vi "host.vi"() -> ()   [LabVIEW 2020]
uses:
  <vilib>/Analysis/baseanly.llb/Vector x A.vi
  <vilib>/Analysis/baseanly.llb/Real Dot Product.vi
  <vilib>/Analysis/Matrix/Numeric/Conversions/Array To Matrix - RA2.vi
  <vilib>/FPGAPlugInAG/cRIO-9054/niLvFpga_Open_cRIO-9054.vi
  <vilib>/rvi/interface/common/dynamic/niFpgaDynamicAddResources.vi
  <vilib>/Utility/error.llb/Error Cluster From Error Code.vi
  <vilib>/rvi/errors/niLvFpgaAdjustHostInterfaceError.vi
  <vilib>/FPGAPlugInAG/Dynamic/niLvFpga_Run_Dynamic.vi
  <vilib>/FPGAPlugInAG/Dynamic/niLvFpga_Close_Dynamic.vi
  <vilib>/rvi/interface/nirviOpenFPGA/nirviOpenFPGA.xnode
  FPGA Bitfiles/mlpsizing_FPGATarget_target_1fQeBnJI5tw.lvbitx
  target.vi
  <vilib>/rvi/interface/nirviMethod/nirviMethod.xnode
  <vilib>/rvi/interface/nirviReadWriteControl/nirviReadWriteControl.xnode
  <vilib>/rvi/interface/nirviCloseFPGA/nirviCloseFPGA.xnode
  <vilib>/Analysis/NI_AALBase.lvlib
  <vilib>/Analysis/Matrix/NI_Matrix.lvlib
  <vilib>/FPGAPlugInAG/Dynamic/niLvFpga_WriteFifo_Dynamic.vi
  <vilib>/rvi/errors/niLvFpgaMergeErrorWithErrorCode.vi
  NiFpgaLv.dll
  <vilib>/rvi/interface/Simulation/niFpgaSimulationCallBeginRW.vi
panel:
  out "clock ticks":u32
  out "error":dbl
  out "y (CPU)":dbl
  out "y (FPGA)":fxp<+/-,33,17>
  out "subarray":fxp<+/-,32,16>[](array[numeric])
  out "V' x A 2":dbl[](array[numeric])
  out "Waveform Graph":waveform(dbl)(graph)
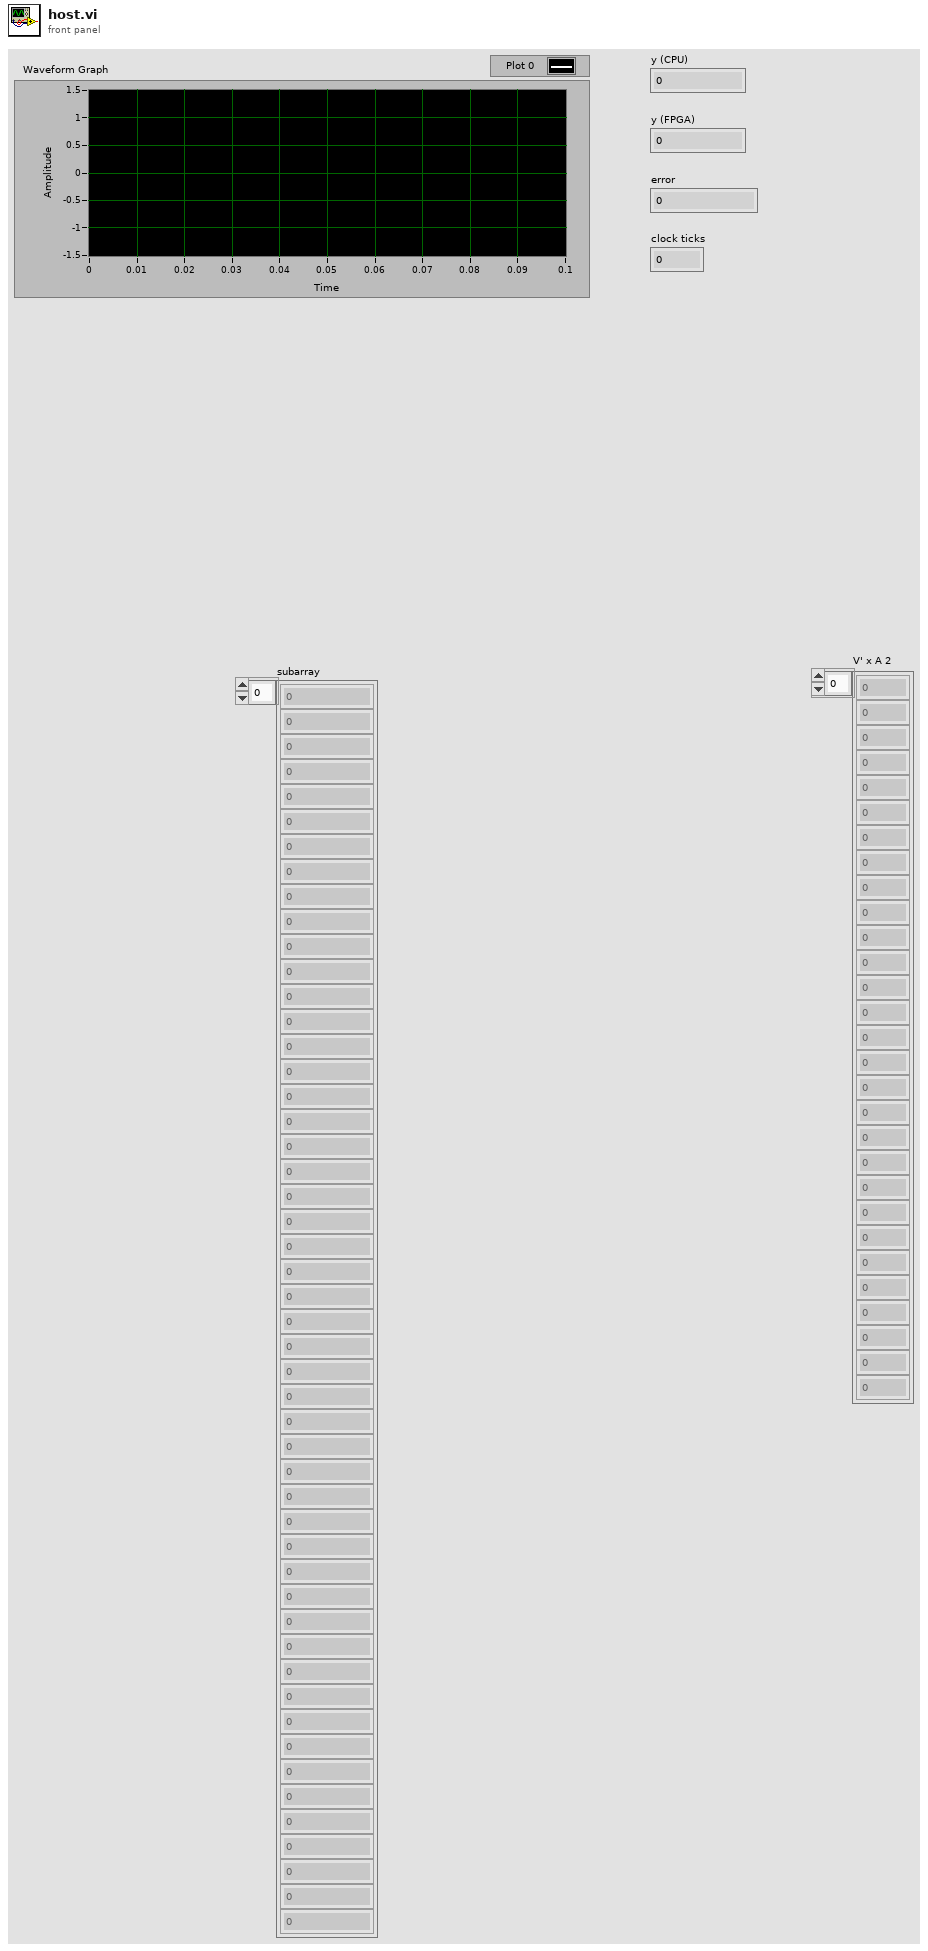
[diagram p1: front panel]
types:
  T1 = typedef "NI_Matrix.lvlib/RealMatrix.ctl" = dbl[][]
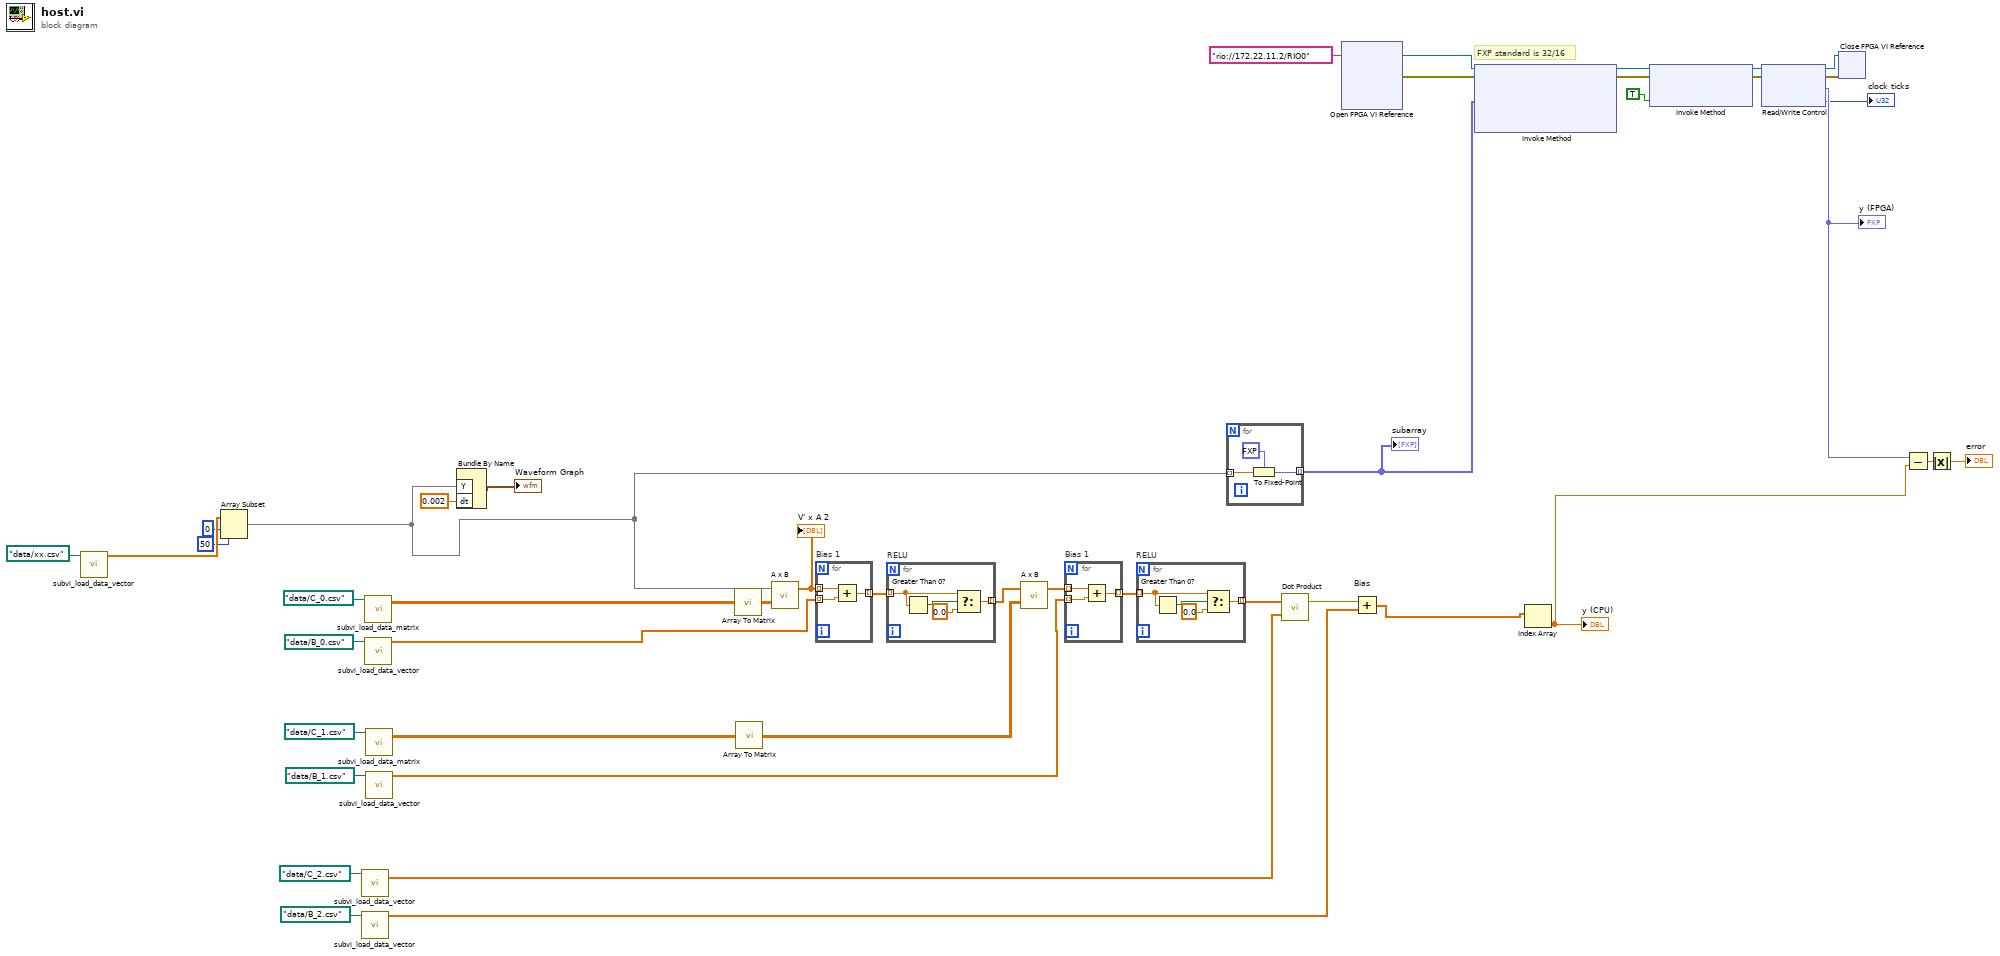
[diagram p0: block diagram]
diagram:
  # "FXP standard is 32/16"
  n1 = call "subvi_load_data_vector.vi"("default name"=path "data/xx.csv") -> ("array type (2D Dbl) out"=w19:dbl[])  [unwired: 10 in]
  n2 = Array Subset(array=w19, index=0, length=50) -> (w18:dbl[])
  n3 = call "subvi_load_data_vector.vi"("default name"=path "data/C_2.csv") -> ("array type (2D Dbl) out"=w28:dbl[])  [unwired: 10 in]
  n4 = call "subvi_load_data_vector.vi"("default name"=path "data/B_2.csv") -> ("array type (2D Dbl) out"=w29:dbl[])  [unwired: 10 in]
  n5 = call "subvi_load_data_matrix.vi"("default name"=path "data/C_0.csv") -> ("array"=w31:dbl[][])  [unwired: 10 in]
  n6 = call "subvi_load_data_vector.vi"("default name"=path "data/B_0.csv") -> ("array type (2D Dbl) out"=w30:dbl[])  [unwired: 10 in]
  n7 = call "subvi_load_data_matrix.vi"("default name"=path "data/C_1.csv") -> ("array"=w6:dbl[][])  [unwired: 10 in]
  n8 = call "subvi_load_data_vector.vi"("default name"=path "data/B_1.csv") -> ("array type (2D Dbl) out"=w5:dbl[])  [unwired: 10 in]
  n9 = Bundle By Name("Y"=w18, "dt"=0.002) -> (→"Waveform Graph":waveform(dbl))  [unwired: 1 in]
  n10 = call-poly <vilib>:"Array To Matrix.vi"("Real 2D Array"=w31) -> ("Real Matrix"=w25:T1)
  n11 = call-poly <vilib>:"Array To Matrix.vi"("Real 2D Array"=w6) -> ("Real Matrix"=w4:T1)
  n12 = call-poly <vilib>:"A x B.vi"("Matrix A"=w25, "Vector V'"=w18) -> ("V' x A"=w39:dbl[])  [unwired: 1 out]
  "V' x A 2" <- w39
  n13 = for "Bias 1" {
    tunnel: w39 -> [w48] mode=indexing
    tunnel: [w47] -> w38 mode=indexing
    tunnel: w30 -> [w46] mode=indexing
    n14 = Add(x=w48, y=w46) -> (x+y=w47:dbl)
  }
  n15 = for "RELU" {
    tunnel: w38 -> [w52] mode=indexing
    tunnel: [w51] -> w3 mode=indexing
    n16 = Greater Than 0?(x=w52) -> (x > 0?=w49:bool)
    n17 = Select(t=w52, s=w49, f=0.0) -> (s? t:f=w51:dbl)
  }
  n18 = call-poly <vilib>:"A x B.vi"("Matrix A"=w4, "Vector V'"=w3) -> ("V' x A"=w1:dbl[])  [unwired: 1 out]
  n19 = for "Bias 1" {
    tunnel: w1 -> [w55] mode=indexing
    tunnel: [w54] -> w9 mode=indexing
    tunnel: w5 -> [w53] mode=indexing
    n20 = Add(x=w55, y=w53) -> (x+y=w54:dbl)
  }
  n21 = for "RELU" {
    tunnel: w9 -> [w59] mode=indexing
    tunnel: [w58] -> w2 mode=indexing
    n22 = Greater Than 0?(x=w59) -> (x > 0?=w56:bool)
    n23 = Select(t=w59, s=w56, f=0.0) -> (s? t:f=w58:dbl)
  }
  n24 = for {
    tunnel: w18 -> [w61] mode=indexing
    tunnel: [w60] -> w24 mode=indexing
    n25 = To Fixed-Point(fixed-point type=fxp<+/-,32,16> 0.0 ("fixed-point"), number=w61) -> (fixed-point=w60:fxp<+/-,32,16>)
  }
  "subarray" <- w24
  n26 = call-poly <vilib>:"Dot Product.vi"("Y Vector"=w28, "X Vector"=w2) -> ("X * Y"=w37:dbl)  [unwired: 1 out]
  n27 = xnode "Open FPGA VI Reference"("resource name"=tag "rio://172.22.11.2/RIO0") -> ("FPGA VI Reference Out"=w45:refnum<k20>, "error out"=w44:errorcluster)  [unwired: 1 in]
  n28 = Add "Bias"(x=w37, y=w29) -> (x+y=w13:dbl[])
  n29 = xnode "Invoke Method"("FPGA VI Reference In"=w45, "error in"=w44, "Data"=w24) -> ("FPGA VI Reference Out"=w27:refnum<k20>, "error out"=w26:errorcluster)  [unwired: 1 in, 1 out]
  n30 = Index Array(array=w13) -> (element=w12:dbl)  [unwired: 1 in]
  "y (CPU)" <- w12
  n31 = xnode "Invoke Method"("FPGA VI Reference In"=w27, "error in"=w26, "Wait Until Done (F)"=TRUE) -> ("FPGA VI Reference Out"=w23:refnum<k20>, "error out"=w22:errorcluster)
  n32 = xnode "Read/Write Control"("FPGA VI Reference In"=w23, "error in"=w22) -> ("FPGA VI Reference Out"=w21:refnum<k20>, "error out"=w20:errorcluster, "y"=w14:fxp<+/-,33,17>, "clock ticks"=→"clock ticks":u32)
  "y (FPGA)" <- w14
  n33 = xnode "Close FPGA VI Reference"("FPGA VI Reference In"=w21, "error in"=w20) -> ()  [unwired: 1 out]
  n34 = Subtract(x=w14, y=w12) -> (x-y=w15:dbl)
  n35 = Absolute Value(x=w15) -> (abs(x)=→"error":dbl)
